vi "ELVIS III v1.0 Reset FPGA.vi"(8 "error in (no error)":errorcluster, 11 "Generic FPGA Reference in":T1) -> (0 "error out":errorcluster, 3 "Generic FPGA Reference out":T1)   [LabVIEW 2021]
uses:
  <vilib>/myRIO/Common/Instrument Driver Framework/Utilities/typedefs/Generic FPGA Reference.ctl
  <vilib>/myRIO/Common/Instrument Driver Framework/ELVIS III v1.0/Resource Manager/typedefs/ELVIS III v1.0 RIO Session Map Action.ctl
  <vilib>/myRIO/Common/Instrument Driver Framework/ELVIS III v1.0/AO Block/typedefs/ELVIS III AO Block Channels FPGA Reference.ctl
  <vilib>/myRIO/Common/Instrument Driver Framework/Utilities/typedefs/myRIO v1.0 Reference.ctl
  <vilib>/myRIO/Common/Instrument Driver Framework/myRIO v1.0/DIO/typedefs/DIO Channels Enum.ctl
  <vilib>/myRIO/Common/Instrument Driver Framework/myRIO v1.0/DI Block/typedefs/DI Block Channels Enum.ctl
  <vilib>/myRIO/Common/Instrument Driver Framework/myRIO v1.0/DO Block/typedefs/DO Block Channels Enum.ctl
  <vilib>/myRIO/Common/Instrument Driver Framework/myRIO v1.0/PWM/typedefs/PWM Channels Enum.ctl
  <vilib>/myRIO/Common/Instrument Driver Framework/myRIO v1.0/Encoder/typedefs/Encoder Channels Enum.ctl
  <vilib>/myRIO/Common/Instrument Driver Framework/myRIO v1.0/SPI/typedefs/SPI Channels Enum.ctl
  <vilib>/myRIO/Common/Instrument Driver Framework/myRIO v1.0/I2C/typedefs/I2C Channels Enum.ctl
  <vilib>/myRIO/Common/Instrument Driver Framework/ELVIS III v1.0/Resource Manager/vis/ELVIS III v1.0 Create Configuration List.vi
  <vilib>/Utility/error.llb/Error Cluster From Error Code.vi
  <vilib>/rvi/errors/niLvFpgaAdjustHostInterfaceError.vi
  <vilib>/rvi/interface/nirviReadWriteControl/nirviReadWriteControl.xnode
  <vilib>/rvi/interface/nirviMethod/nirviMethod.xnode
  <vilib>/rvi/interface/Simulation/niFpgaSimulationCallBeginRW.vi
  <vilib>/rvi/errors/niLvFpgaMergeErrorWithErrorCode.vi
  <vilib>/FPGAPlugInAG/Dynamic/niLvFpga_StartFifo_Dynamic.vi
  <vilib>/FPGAPlugInAG/Dynamic/niLvFpga_StopFifo_Dynamic.vi
  NiFpgaLv.dll
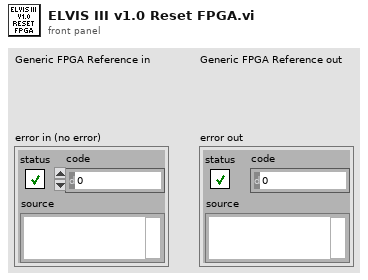
[diagram p1: front panel]
types:
  T1 = typedef "Generic FPGA Reference.ctl" = refnum<k20>
  T2 = typedef "ELVIS III v1.0 RIO Session Map Action.ctl" = enum16{"Add Session", "Remove Session", "Get Active Sessions", "Get Owning Sessions"}
  T3 = typedef "myRIO v1.0 Reference.ctl" = cluster{"Generic FPGA Reference":T1, "Allow multiple opens":bool}
  T4 = typedef "DIO Channels Enum.ctl" = enum16{"Not Connected", "C/DIO0", "C/DIO1", "C/DIO2", "C/DIO3", "C/DIO4", "C/DIO5", "C/DIO6", "C/DIO7", "A/DIO0", "A/DIO1", "A/DIO2", "A/DIO3", "A/DIO4", "A/DIO5", "A/DIO6", "A/DIO7", "A/DIO8", "A/DIO9", "A/DIO10", "A/DIO11", "A/DIO12", "A/DIO13", "A/DIO14", "A/DIO15", "A/DIO16", "A/DIO17", "A/DIO18", "A/DIO19", "B/DIO0", "B/DIO1", "B/DIO2", "B/DIO3", "B/DIO4", "B/DIO5", "B/DIO6", "B/DIO7", "B/DIO8", "B/DIO9", "B/DIO10", "B/DIO11", "B/DIO12", "B/DIO13", "B/DIO14", "B/DIO15", "B/DIO16", "B/DIO17", "B/DIO18", "B/DIO19", "LED0", "LED1", "LED2", "LED3", "Button0", "DIO/DIO0", "DIO/DIO1", "DIO/DIO2", "DIO/DIO3", "DIO/DIO4", "DIO/DIO5", "DIO/DIO6", "DIO/DIO7", "DIO/DIO8", "DIO/DIO9", "SPI/CS0", "SPI/CS1", "SPI/CS2", "SPI/CS3", "LED RADIO (Green)", "LED RADIO (Red)", "LED COMM (Green)", "LED COMM (Red)", "LED MODE (Green)", "LED MODE (Red)"}
  T5 = typedef "DI Block Channels Enum.ctl" = enum16{"Not Connected", "A/DI0 (N Samples)", "A/DI1 (N Samples)", "A/DI2 (N Samples)", "A/DI3 (N Samples)", "A/DI4 (N Samples)", "A/DI5 (N Samples)", "A/DI6 (N Samples)", "A/DI7 (N Samples)", "A/DI8 (N Samples)", "A/DI9 (N Samples)", "A/DI10 (N Samples)", "A/DI11 (N Samples)", "A/DI12 (N Samples)", "A/DI13 (N Samples)", "A/DI14 (N Samples)", "A/DI15 (N Samples)", "A/DI16 (N Samples)", "A/DI17 (N Samples)", "A/DI18 (N Samples)", "A/DI19 (N Samples)", "B/DI0 (N Samples)", "B/DI1 (N Samples)", "B/DI2 (N Samples)", "B/DI3 (N Samples)", "B/DI4 (N Samples)", "B/DI5 (N Samples)", "B/DI6 (N Samples)", "B/DI7 (N Samples)", "B/DI8 (N Samples)", "B/DI9 (N Samples)", "B/DI10 (N Samples)", "B/DI11 (N Samples)", "B/DI12 (N Samples)", "B/DI13 (N Samples)", "B/DI14 (N Samples)", "B/DI15 (N Samples)", "B/DI16 (N Samples)", "B/DI17 (N Samples)", "B/DI18 (N Samples)", "B/DI19 (N Samples)"}
  T6 = typedef "DO Block Channels Enum.ctl" = enum16{"Not Connected", "A/DO0 (N Samples)", "A/DO1 (N Samples)", "A/DO2 (N Samples)", "A/DO3 (N Samples)", "A/DO4 (N Samples)", "A/DO5 (N Samples)", "A/DO6 (N Samples)", "A/DO7 (N Samples)", "A/DO8 (N Samples)", "A/DO9 (N Samples)", "A/DO10 (N Samples)", "A/DO11 (N Samples)", "A/DO12 (N Samples)", "A/DO13 (N Samples)", "A/DO14 (N Samples)", "A/DO15 (N Samples)", "A/DO16 (N Samples)", "A/DO17 (N Samples)", "A/DO18 (N Samples)", "A/DO19 (N Samples)", "B/DO0 (N Samples)", "B/DO1 (N Samples)", "B/DO2 (N Samples)", "B/DO3 (N Samples)", "B/DO4 (N Samples)", "B/DO5 (N Samples)", "B/DO6 (N Samples)", "B/DO7 (N Samples)", "B/DO8 (N Samples)", "B/DO9 (N Samples)", "B/DO10 (N Samples)", "B/DO11 (N Samples)", "B/DO12 (N Samples)", "B/DO13 (N Samples)", "B/DO14 (N Samples)", "B/DO15 (N Samples)", "B/DO16 (N Samples)", "B/DO17 (N Samples)", "B/DO18 (N Samples)", "B/DO19 (N Samples)"}
  T7 = typedef "PWM Channels Enum.ctl" = enum16{"Not Connected", "C/PWM0", "C/PWM1", "A/PWM0", "A/PWM1", "A/PWM2", "A/PWM3", "A/PWM4", "A/PWM5", "A/PWM6", "A/PWM7", "A/PWM8", "A/PWM9", "A/PWM10", "A/PWM11", "A/PWM12", "A/PWM13", "A/PWM14", "A/PWM15", "A/PWM16", "A/PWM17", "A/PWM18", "A/PWM19", "B/PWM0", "B/PWM1", "B/PWM2", "B/PWM3", "B/PWM4", "B/PWM5", "B/PWM6", "B/PWM7", "B/PWM8", "B/PWM9", "B/PWM10", "B/PWM11", "B/PWM12", "B/PWM13", "B/PWM14", "B/PWM15", "B/PWM16", "B/PWM17", "B/PWM18", "B/PWM19", "PWM/PWM0", "PWM/PWM1", "PWM/PWM2", "PWM/PWM3", "PWM/PWM4", "PWM/PWM5", "PWM/PWM6", "PWM/PWM7", "PWM/PWM8", "PWM/PWM9"}
  T8 = typedef "Encoder Channels Enum.ctl" = enum16{"Not Connected", "C/ENC0", "C/ENC1", "A/ENC", "A/ENC0", "A/ENC1", "A/ENC2", "A/ENC3", "A/ENC4", "A/ENC5", "A/ENC6", "A/ENC7", "A/ENC8", "A/ENC9", "B/ENC", "B/ENC0", "B/ENC1", "B/ENC2", "B/ENC3", "B/ENC4", "B/ENC5", "B/ENC6", "B/ENC7", "B/ENC8", "B/ENC9", "DIO/ENC0", "DIO/ENC1", "DIO/ENC2", "DIO/ENC3", "DIO/ENC4"}
  T9 = typedef "SPI Channels Enum.ctl" = enum16{"Not Connected", "A/SPI", "B/SPI", "SPI/SPI"}
  T10 = typedef "I2C Channels Enum.ctl" = enum16{"Not Connected", "A/I2C", "B/I2C", "I2C/I2C"}
  T11 = cluster{"Session":u32, "Channel Names":string[]}[]
  T12 = typedef "ELVIS III AO Block Channels FPGA Reference.ctl" = refnum<k20>
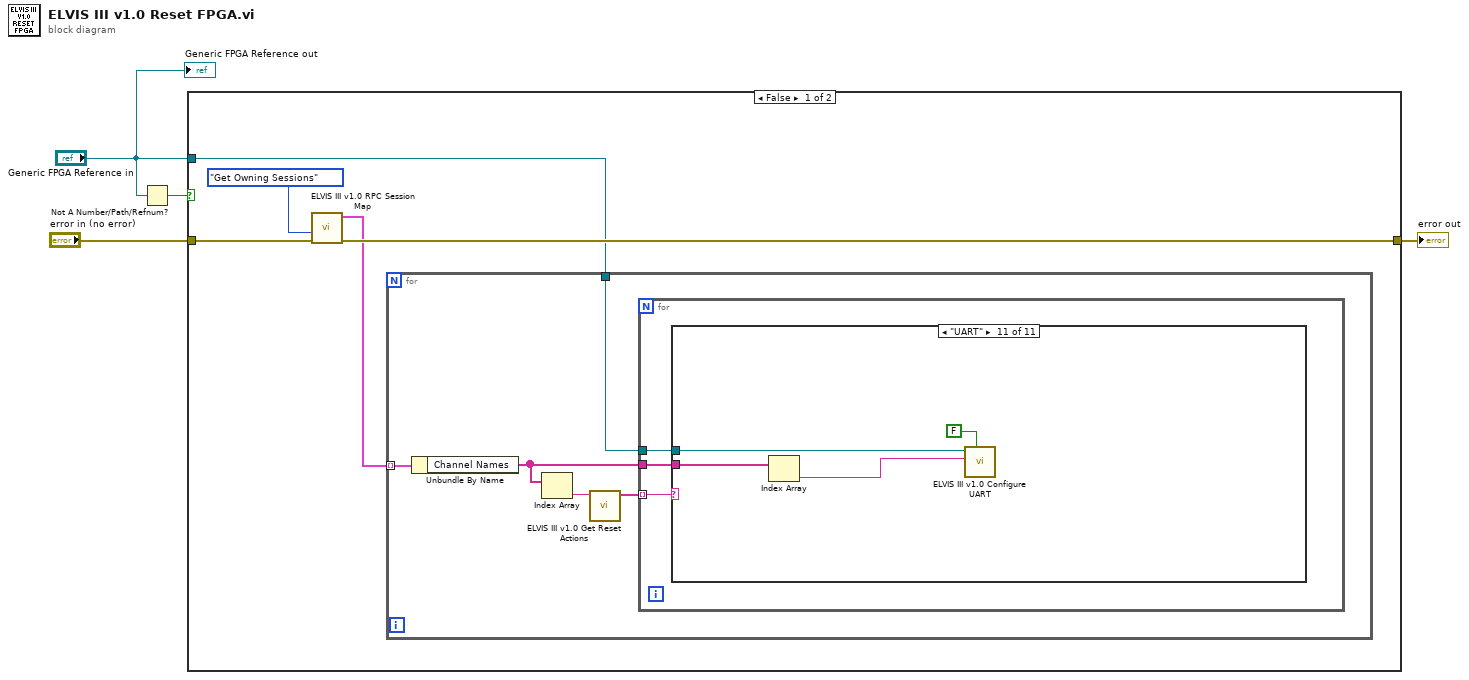
[diagram p0: block diagram]
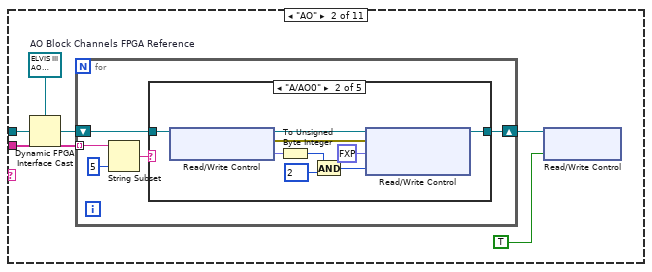
[diagram p3: hidden frame]
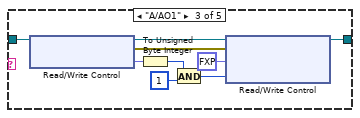
[diagram p5: hidden frame]
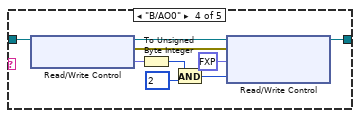
[diagram p6: hidden frame]
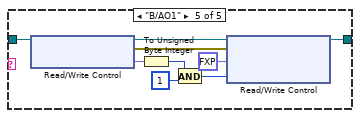
[diagram p7: hidden frame]
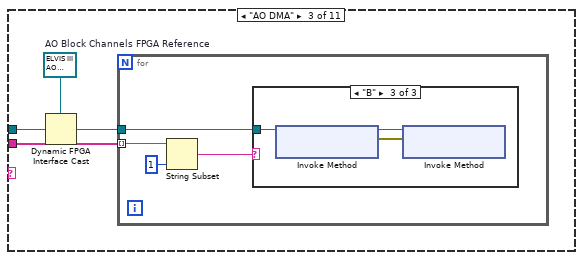
[diagram p8: hidden frame]
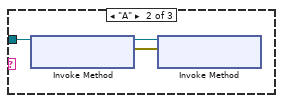
[diagram p10: hidden frame]
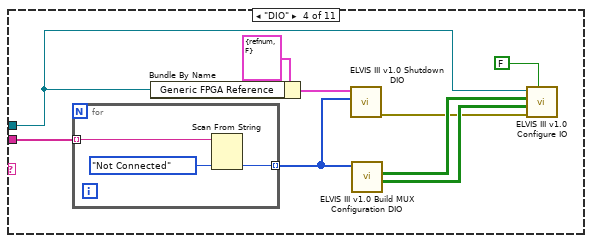
[diagram p11: hidden frame]
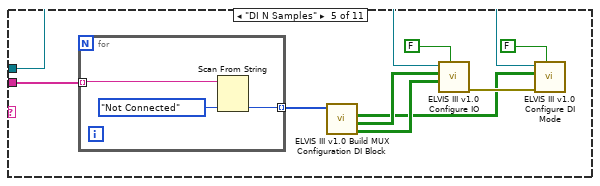
[diagram p12: hidden frame]
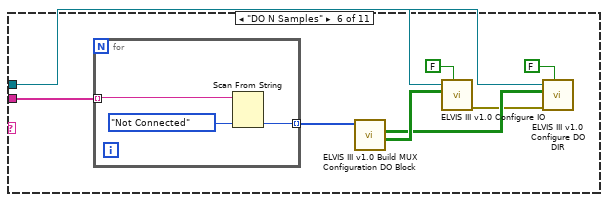
[diagram p13: hidden frame]
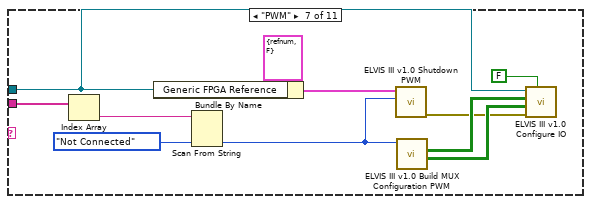
[diagram p14: hidden frame]
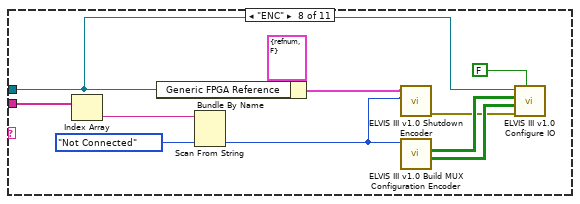
[diagram p15: hidden frame]
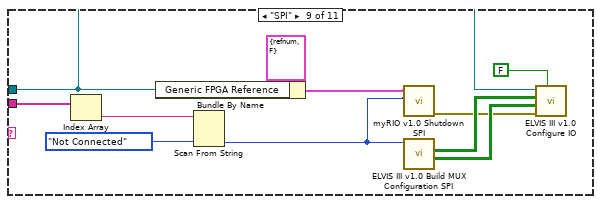
[diagram p16: hidden frame]
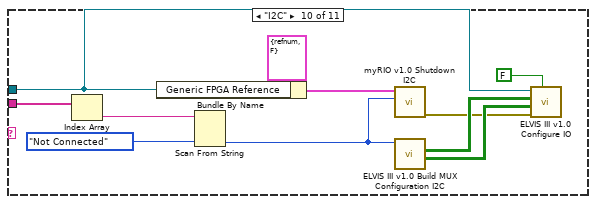
[diagram p17: hidden frame]
diagram:
  n1 = Not A Number/Path/Refnum?(number/path/refnum="Generic FPGA Reference in") -> (NaN/Path/Refnum?=w3:bool)
  n2 = case shown="False" w3 {
    tunnel: "Generic FPGA Reference in" -> [w5 _]
    tunnel: [w7 w163] -> w4
    tunnel: "error in (no error)" -> [w8 w163]
    frame False {
      n3 = call <vilib>:"ELVIS III v1.0 RPC Session Map.vi"("error in (no error)"=w8, "Action"=ELVIS_III_v1.0_RIO_Session_Map_Action."Get Owning Sessions") -> ("error out"=w7:errorcluster, "Session Infos"=w6:T11)  [unwired: 8 in]
      n4 = for {
        tunnel: w6 -> [w14] mode=indexing
        tunnel: w5 -> [w10]
        n5 = Unbundle By Name(w14) -> ("Channel Names"=w13:string[])
        n6 = Index Array(array=w13) -> (element=w12:string)  [unwired: 1 in]
        n7 = call <vilib>:"ELVIS III v1.0 Get Reset Actions.vi"("String"=w12) -> ("Resources"=w11:string[])  [unwired: 9 in, 1 out]
        n8 = for {
          tunnel: w13 -> [w17]
          tunnel: w11 -> [w16] mode=indexing
          tunnel: w10 -> [w15]
          n9 = case shown="\"UART\"" w16 {
            tunnel: w17 -> [_ w23 w69 w88 w100 w111 w125 w134 w141 w152 w162]
            tunnel: w15 -> [_ w19 w68 w81 w94 w105 w117 w126 w140 w151 w160]
            frame "No", Default {
            }
            frame "AO" {
              w20 = T12 refnum  # AO Block Channels FPGA Reference
              n10 = Dynamic FPGA Interface Cast(Session In=w20, Type=w19) -> (Session Out=w18:T12)
              n11 = for {
                tunnel: w23 -> [w27] mode=indexing
                shift-right: [w24] -> w22
                shift-left: w18 -> [w28]
                n12 = String Subset(string=w27, length (rest)=5 ("length (rest)")) -> (substring=w26:string)  [unwired: 1 in]
                n13 = case shown="\"A/AO0\"" w26 {
                  tunnel: w28 -> [w29 w37 w41 w50 w59]
                  tunnel: [w29 w31 w40 w49 w58] -> w24
                  frame "None", Default {
                  }
                  frame "A/AO0" {
                    n14 = xnode "Read/Write Control"("FPGA VI Reference In"=w37) -> ("FPGA VI Reference Out"=w36:T12, "error out"=w30:errorcluster, "AO.A.DMA_ENA"=w35:fxp<+,2,2>)  [unwired: 1 in]
                    n15 = To Unsigned Byte Integer(number=w35) -> (unsigned 8bit integer=w33:u8)
                    n16 = And(x=w33, y=u8 2) -> (x .and. y?=w34:u8)
                    n17 = xnode "Read/Write Control"("FPGA VI Reference In"=w36, "error in"=w30, "AO.A_0.VAL"=fxp<+/-,20,5> 0.0, "AO.A.DMA_ENA"=w34) -> ("FPGA VI Reference Out"=w31:T12)  [unwired: 1 out]
                  }
                  frame "A/AO1" {
                    n18 = xnode "Read/Write Control"("FPGA VI Reference In"=w41) -> ("FPGA VI Reference Out"=w44:T12, "error out"=w39:errorcluster, "AO.A.DMA_ENA"=w45:fxp<+,2,2>)  [unwired: 1 in]
                    n19 = To Unsigned Byte Integer(number=w45) -> (unsigned 8bit integer=w47:u8)
                    n20 = And(x=w47, y=u8 1) -> (x .and. y?=w46:u8)
                    n21 = xnode "Read/Write Control"("FPGA VI Reference In"=w44, "error in"=w39, "AO.A_1.VAL"=fxp<+/-,20,5> 0.0 ("AO.A_0.VAL"), "AO.A.DMA_ENA"=w46) -> ("FPGA VI Reference Out"=w40:T12)  [unwired: 1 out]
                  }
                  frame "B/AO0" {
                    n22 = xnode "Read/Write Control"("FPGA VI Reference In"=w50) -> ("FPGA VI Reference Out"=w55:T12, "error out"=w48:errorcluster, "AO.B.DMA_ENA"=w54:fxp<+,2,2>)  [unwired: 1 in]
                    n23 = To Unsigned Byte Integer(number=w54) -> (unsigned 8bit integer=w52:u8)
                    n24 = And(x=w52, y=u8 2) -> (x .and. y?=w53:u8)
                    n25 = xnode "Read/Write Control"("FPGA VI Reference In"=w55, "error in"=w48, "AO.B_0.VAL"=fxp<+/-,20,5> 0.0 ("AO.A_0.VAL"), "AO.B.DMA_ENA"=w53) -> ("FPGA VI Reference Out"=w49:T12)  [unwired: 1 out]
                  }
                  frame "B/AO1" {
                    n26 = xnode "Read/Write Control"("FPGA VI Reference In"=w59) -> ("FPGA VI Reference Out"=w62:T12, "error out"=w57:errorcluster, "AO.B.DMA_ENA"=w63:fxp<+,2,2>)  [unwired: 1 in]
                    n27 = To Unsigned Byte Integer(number=w63) -> (unsigned 8bit integer=w65:u8)
                    n28 = And(x=w65, y=u8 1) -> (x .and. y?=w64:u8)
                    n29 = xnode "Read/Write Control"("FPGA VI Reference In"=w62, "error in"=w57, "AO.B_1.VAL"=fxp<+/-,20,5> 0.0 ("AO.A_0.VAL"), "AO.B.DMA_ENA"=w64) -> ("FPGA VI Reference Out"=w58:T12)  [unwired: 1 out]
                  }
                }
              }
              n30 = xnode "Read/Write Control"("FPGA VI Reference In"=w22, "AO.SYS.GO"=TRUE) -> ()  [unwired: 1 in, 2 out]
            }
            frame "AO DMA" {
              w67 = T12 refnum  # AO Block Channels FPGA Reference
              n31 = Dynamic FPGA Interface Cast(Session In=w67, Type=w68) -> (Session Out=w66:T12)
              n32 = for {
                tunnel: w69 -> [w73] mode=indexing
                tunnel: w66 -> [w71]
                n33 = String Subset(string=w73, length (rest)=1 ("length (rest)")) -> (substring=w70:string)  [unwired: 1 in]
                n34 = case shown="\"B\"" w70 {
                  tunnel: w71 -> [_ w74 w77]
                  frame "None", Default {
                  }
                  frame "A" {
                    n35 = xnode "Invoke Method"("FPGA VI Reference In"=w74) -> ("FPGA VI Reference Out"=w76:T12, "error out"=w75:errorcluster)  [unwired: 1 in]
                    n36 = xnode "Invoke Method"("FPGA VI Reference In"=w76, "error in"=w75) -> ()  [unwired: 2 out]
                  }
                  frame "B" {
                    n37 = xnode "Invoke Method"("FPGA VI Reference In"=w77) -> ("FPGA VI Reference Out"=w78:T12, "error out"=w79:errorcluster)  [unwired: 1 in]
                    n38 = xnode "Invoke Method"("FPGA VI Reference In"=w78, "error in"=w79) -> ()  [unwired: 2 out]
                  }
                }
              }
            }
            frame "DIO" {
              n39 = for {
                tunnel: w88 -> [w90] mode=indexing
                tunnel: [w89] -> w82 mode=indexing
                n40 = Scan From String(input string=w90, default 1=DIO_Channels_Enum."Not Connected" ("Channel")) -> (output 1=w89:T4)  [unwired: 3 in, 3 out]
              }
              n41 = Bundle By Name(cluster=T3 {"Generic FPGA Reference"=refnum, "Allow multiple opens"=FALSE} ("myRIO Ref In"), "Generic FPGA Reference"=w81) -> (w86:T3)
              n42 = call <vilib>:"ELVIS III v1.0 Shutdown DIO.vi"("Channel List"=w82, "myRIO Ref In"=w86) -> ("error out"=w80:errorcluster)  [unwired: 8 in, 1 out]
              n43 = call <vilib>:"ELVIS III v1.0 Build MUX Configuration DIO.vi"("DIO Channel List"=w82) -> ("Configuration Bitmask Array"=w83:bool[][], "Configration Bitcode Array"=w84:bool[][])  [unwired: 8 in, 1 out]
              n44 = call <vilib>:"ELVIS III v1.0 Configure IO.vi"("Value"=FALSE ("Clear?"), "error in (no error)"=w80, "Bitmask Array"=w83, "Bitcode Array"=w84, "myRIO FPGA Ref In"=w81) -> ()  [unwired: 6 in, 1 out]
            }
            frame "DI N Samples" {
              n45 = for {
                tunnel: w100 -> [w103] mode=indexing
                tunnel: [w102] -> w95 mode=indexing
                n46 = Scan From String(input string=w103, default 1=DI_Block_Channels_Enum."Not Connected" ("DI Block Read Channels Enum")) -> (output 1=w102:T5)  [unwired: 3 in, 3 out]
              }
              n47 = call <vilib>:"ELVIS III v1.0 Build MUX Configuration DI Block.vi"("DI (N Samples) Channel List"=w95) -> ("Configuration Bitmask Array"=w98:bool[][], "Configration Bitcode Array"=w99:bool[][], "DIO Mode Bitask"=w92:bool[][])  [unwired: 7 in, 1 out]
              n48 = call <vilib>:"ELVIS III v1.0 Configure IO.vi"("Value"=FALSE, "Bitmask Array"=w98, "Bitcode Array"=w99, "myRIO FPGA Ref In"=w94) -> ("error out"=w93:errorcluster)  [unwired: 7 in]
              n49 = call <vilib>:"ELVIS III v1.0 Configure DI Mode.vi"("Apply Bitmask?"=FALSE ("Set or Reset?"), "error in (no error)"=w93, "Bitmask Array"=w92, "myRIO FPGA Ref In"=w94) -> ()  [unwired: 7 in, 1 out]
            }
            frame "DO N Samples" {
              n50 = for {
                tunnel: w111 -> [w114] mode=indexing
                tunnel: [w113] -> w104 mode=indexing
                n51 = Scan From String(input string=w114, default 1=DO_Block_Channels_Enum."Not Connected" ("DO Block Write Channels Enum")) -> (output 1=w113:T6)  [unwired: 3 in, 3 out]
              }
              n52 = call <vilib>:"ELVIS III v1.0 Build MUX Configuration DO Block.vi"("DO (N Samples) Channel List"=w104) -> ("Configration Bitcode Array"=w109:bool[][], "DIO Mode Bitmask"=w107:bool[][])  [unwired: 7 in, 2 out]
              n53 = call <vilib>:"ELVIS III v1.0 Configure IO.vi"("Value"=FALSE, "Bitcode Array"=w109, "myRIO FPGA Ref In"=w105) -> ("error out"=w106:errorcluster)  [unwired: 8 in]
              n54 = call <vilib>:"ELVIS III v1.0 Configure DO DIR.vi"("Apply Bitmask?"=FALSE, "error in (no error)"=w106, "Bitmask Array"=w107, "myRIO FPGA Ref In"=w105) -> ()  [unwired: 7 in, 1 out]
            }
            frame "PWM" {
              n55 = Index Array(array=w125) -> (element=w123:string)  [unwired: 1 in]
              n56 = Bundle By Name(cluster=T3 {"Generic FPGA Reference"=refnum, "Allow multiple opens"=FALSE} ("myRIO Ref In"), "Generic FPGA Reference"=w117) -> (w121:T3)
              n57 = Scan From String(input string=w123, default 1=PWM_Channels_Enum."Not Connected" ("PWM Channel")) -> (output 1=w116:T7)  [unwired: 3 in, 3 out]
              n58 = call <vilib>:"ELVIS III v1.0 Shutdown PWM.vi"("Channel"=w116, "myRIO Ref In"=w121) -> ("error out"=w115:errorcluster)  [unwired: 8 in, 1 out]
              n59 = call <vilib>:"ELVIS III v1.0 Build MUX Configuration PWM.vi"("Channel"=w116) -> ("Configuration Bitmask Array"=w118:bool[][], "Configuration BitCode Array"=w119:bool[][])  [unwired: 8 in, 1 out]
              n60 = call <vilib>:"ELVIS III v1.0 Configure IO.vi"("Value"=FALSE ("Clear?"), "error in (no error)"=w115, "Bitmask Array"=w118, "Bitcode Array"=w119, "myRIO FPGA Ref In"=w117) -> ()  [unwired: 6 in, 1 out]
            }
            frame "ENC" {
              n61 = Index Array(array=w134) -> (element=w136:string)  [unwired: 1 in]
              n62 = Bundle By Name(cluster=T3 {"Generic FPGA Reference"=refnum, "Allow multiple opens"=FALSE} ("myRIO Ref In"), "Generic FPGA Reference"=w126) -> (w129:T3)
              n63 = Scan From String(input string=w136, default 1=Encoder_Channels_Enum."Not Connected" ("Encoder Channel")) -> (output 1=w128:T8)  [unwired: 3 in, 3 out]
              n64 = call <vilib>:"ELVIS III v1.0 Shutdown Encoder.vi"("Channel"=w128, "myRIO Ref In"=w129) -> ("error out"=w127:errorcluster)  [unwired: 8 in, 1 out]
              n65 = call <vilib>:"ELVIS III v1.0 Build MUX Configuration Encoder.vi"("Channel"=w128) -> ("Configuration Bitmask Array"=w130:bool[][], "Configuration BitCode Array"=w131:bool[][])  [unwired: 8 in, 1 out]
              n66 = call <vilib>:"ELVIS III v1.0 Configure IO.vi"("Value"=FALSE ("Clear?"), "error in (no error)"=w127, "Bitmask Array"=w130, "Bitcode Array"=w131, "myRIO FPGA Ref In"=w126) -> ()  [unwired: 6 in, 1 out]
            }
            frame "SPI" {
              n67 = Index Array(array=w141) -> (element=w147:string)  [unwired: 1 in]
              n68 = Bundle By Name(cluster=T3 {"Generic FPGA Reference"=refnum, "Allow multiple opens"=FALSE} ("myRIO Ref In"), "Generic FPGA Reference"=w140) -> (w139:T3)
              n69 = Scan From String(input string=w147, default 1=SPI_Channels_Enum."Not Connected" ("SPI Channel")) -> (output 1=w137:T9)  [unwired: 3 in, 3 out]
              n70 = call <vilib>:"myRIO v1.0 Shutdown SPI.vi"("SPI Channel"=w137, "myRIO Ref In"=w139) -> ("error out"=w138:errorcluster)  [unwired: 8 in, 1 out]
              n71 = call <vilib>:"ELVIS III v1.0 Build MUX Configuration SPI.vi"("Channel"=w137) -> ("Configuration Bitmask Array"=w145:bool[][], "Configuration BitCode Array"=w144:bool[][])  [unwired: 8 in, 1 out]
              n72 = call <vilib>:"ELVIS III v1.0 Configure IO.vi"("Value"=FALSE ("Clear?"), "error in (no error)"=w138, "Bitmask Array"=w145, "Bitcode Array"=w144, "myRIO FPGA Ref In"=w140) -> ()  [unwired: 6 in, 1 out]
            }
            frame "I2C" {
              n73 = Index Array(array=w152) -> (element=w158:string)  [unwired: 1 in]
              n74 = Bundle By Name(cluster=T3 {"Generic FPGA Reference"=refnum, "Allow multiple opens"=FALSE} ("myRIO Ref In"), "Generic FPGA Reference"=w151) -> (w150:T3)
              n75 = Scan From String(input string=w158, default 1=I2C_Channels_Enum."Not Connected" ("I2C Channel")) -> (output 1=w149:T10)  [unwired: 3 in, 3 out]
              n76 = call <vilib>:"myRIO v1.0 Shutdown I2C.vi"("Channel"=w149, "myRIO Ref In"=w150) -> ("error out"=w148:errorcluster)  [unwired: 8 in, 1 out]
              n77 = call <vilib>:"ELVIS III v1.0 Build MUX Configuration I2C.vi"("Channel"=w149) -> ("Configuration Bitmask Array"=w154:bool[][], "Configuration BitCode Array"=w155:bool[][])  [unwired: 8 in, 1 out]
              n78 = call <vilib>:"ELVIS III v1.0 Configure IO.vi"("Value"=FALSE ("Clear?"), "error in (no error)"=w148, "Bitmask Array"=w154, "Bitcode Array"=w155, "myRIO FPGA Ref In"=w151) -> ()  [unwired: 6 in, 1 out]
            }
            frame "UART" {
              n79 = Index Array(array=w162) -> (element=w159:string)  [unwired: 1 in]
              n80 = call <vilib>:"ELVIS III v1.0 Configure UART.vi"("Reserve?"=FALSE ("Clear?"), "VISA resource name in"=w159, "myRIO FPGA Ref"=w160) -> ()  [unwired: 8 in, 1 out]
            }
          }
        }
      }
    }
    frame True {
    }
  }
  "error out" <- w4
  "Generic FPGA Reference out" <- "Generic FPGA Reference in"
